vi "SCMP - Waveform int.vi"(8 "error in (no error)":errorcluster, 9 "LCVR Voltages":dbl[][](array[numeric]), 10 "Cycles":i32, 11 "FPS in":dbl) -> (0 "error out":errorcluster, 2 "AO Graph":waveform(dbl)[](array[waveform]), 3 "Refnum out":refnum<k21>, 4 "SCD Waveforms":waveform(dbl)[](graph), 5 "duration":dbl, 6 "COMP Waveforms":waveform(dbl)[](graph), 7 "LCVR Relaxtion Time":dbl)   [LabVIEW 2014]
uses:
  <vilib>/Waveform/WDTOps.llb/WDT Waveform Duration DBL.vi
  <vilib>/DAQmx/create/channels.llb/DAQmx Create Channel (AO-Voltage-Basic).vi
  <vilib>/DAQmx/configure/timing.llb/DAQmx Timing (Use Waveform).vi
  <vilib>/DAQmx/write.llb/DAQmx Write (Analog 1D Wfm NChan NSamp).vi
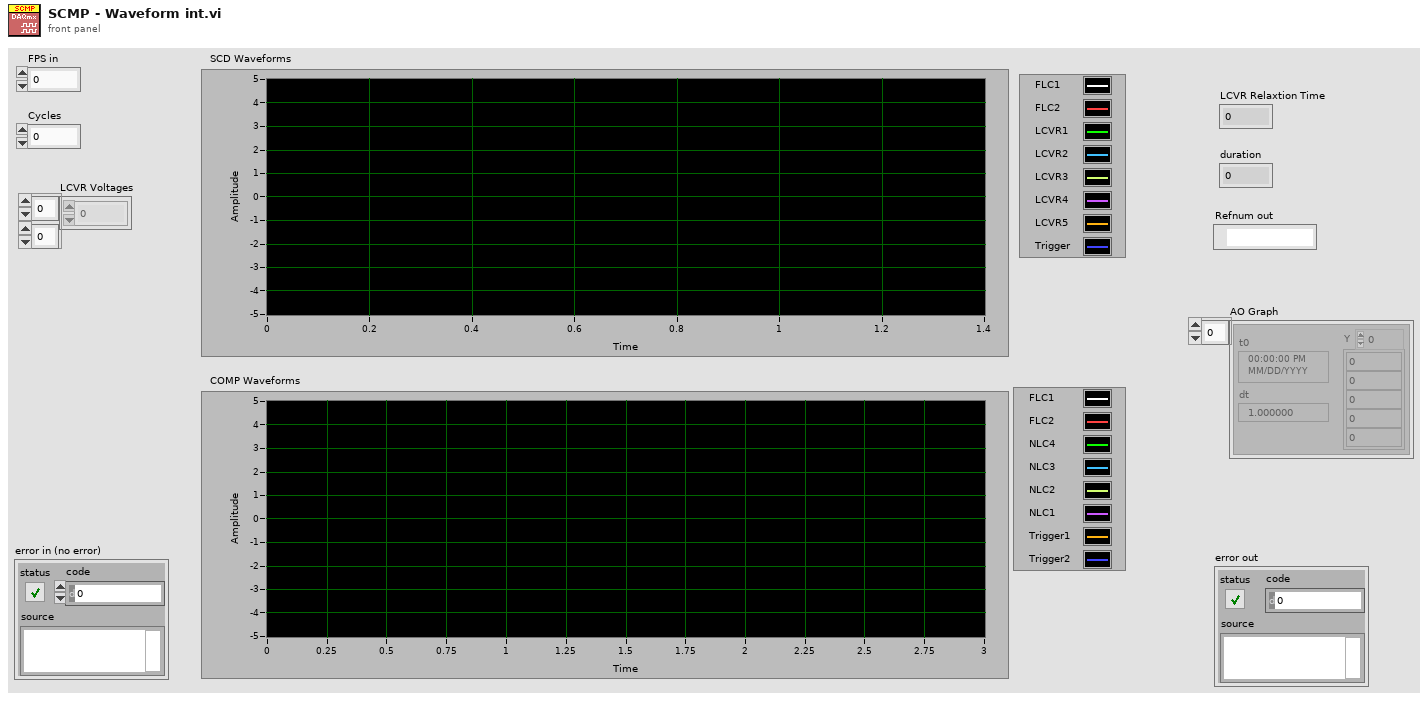
[diagram p1: front panel]
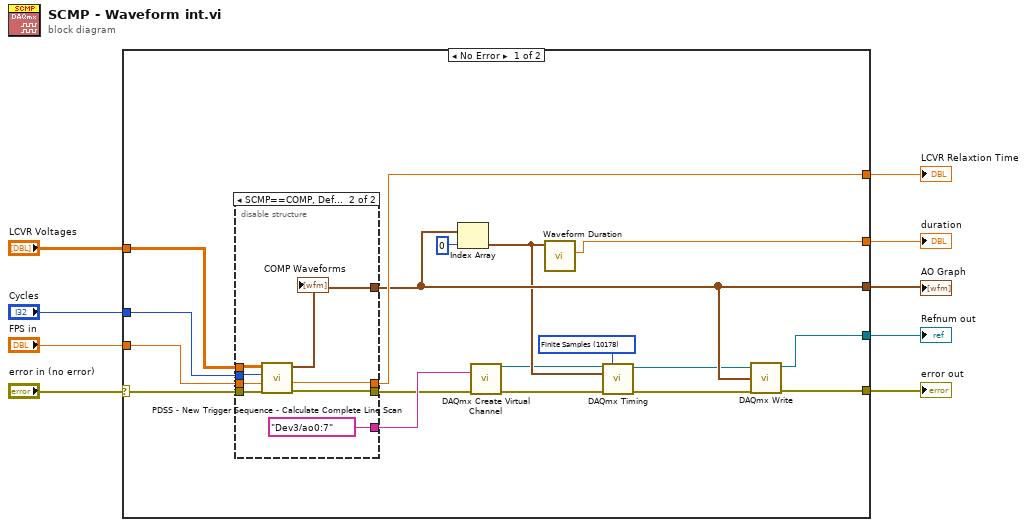
[diagram p0: block diagram]
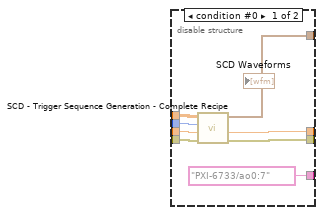
[diagram p2: hidden frame]
diagram:
  n1 = case shown="No Error" "error in (no error)" {
    selector: "error in (no error)" -> [w10 w44]
    tunnel: [w27 _] -> w9
    tunnel: [w26 _] -> w8
    tunnel: "Cycles" -> [w25 _]
    tunnel: "FPS in" -> [w24 _]
    tunnel: [w23 _] -> w5
    tunnel: [w21 _] -> w4
    tunnel: [w20 w44] -> w3
    tunnel: "LCVR Voltages" -> [w19 _]
    frame No Error {
      w11 = 10178 items=["Finite Samples"=10178, "Continuous Samples"=10123] ("sample mode")
      n2 = disable-structure shown="SCMP==COMP, Default" {
        disable-tunnel: [w35 w40] -> w15
        disable-tunnel: w19 -> [w34 w43]
        disable-tunnel: [w29 w38] -> w21
        disable-tunnel: w24 -> [w33 w36]
        disable-tunnel: w10 -> [w32 w41]
        disable-tunnel: [w31 w39] -> w26
        disable-tunnel: w25 -> [w30 w42]
        disable-tunnel: [tag "PXI-6733/ao0:7" ("physical channels") tag "Dev3/ao0:7" ("physical channels")] -> w22
        frame condition #0 {
          n3 = call "SCD - Trigger Sequence Generation - Complete Recipe.vi"("error in"=w32, "FPS"=w33, "Modulation Cycles\nAt Each Wavelength"=w30, "LCVR Voltages"=w34) -> ("error out"=w35:errorcluster, "LCVR Relaxtion Time"=w31:dbl, "SCD Waveforms (Graph)"=w29:waveform(dbl)[])  [unwired: 5 in]
          "SCD Waveforms" <- w29
        }
        frame condition #1 (active) {
          n4 = call "PDSS - New Trigger Sequence - Calculate Complete Line Scan.vi"("error in"=w41, "FPS"=w36, "Modulation Cycles\nAt Each Wavelength"=w42, "LCVR Voltages"=w43) -> ("error out"=w40:errorcluster, "LCVR Relaxtion Time"=w39:dbl, "AO Graph"=w38:waveform(dbl)[])  [unwired: 5 in]
          "COMP Waveforms" <- w38
        }
      }
      n5 = Index Array(array=w21, index=0) -> (element=w18:waveform(dbl))
      n6 = call-poly <vilib>:"DAQmx Create Virtual Channel.vi"("physical channels"=w22, "error in"=w15) -> ("task out"=w13:refnum<k21>, "error out"=w12:errorcluster)  [unwired: 12 in]
      n7 = call-poly <vilib>:"Waveform Duration.vi"("waveform in"=w18) -> ("duration"=w27:dbl)  [unwired: 8 in, 2 out]
      n8 = call-poly <vilib>:"DAQmx Timing.vi"("task/channels in"=w13, "sample mode"=w11, "waveform"=w18, "error in"=w12) -> ("task out"=w17:refnum<k21>, "error out"=w16:errorcluster)  [unwired: 10 in]
      n9 = call-poly <vilib>:"DAQmx Write.vi"("task/channels in"=w17, "data"=w21, "error in"=w16) -> ("task out"=w23:refnum<k21>, "error out"=w20:errorcluster)  [unwired: 10 in, 1 out]
    }
    frame Error {
    }
  }
  "duration" <- w9
  "LCVR Relaxtion Time" <- w8
  "Refnum out" <- w5
  "AO Graph" <- w4
  "error out" <- w3
